vi "Activate License throuch Network.vi"() -> ()   [LabVIEW 2018]
doc: "Demonstrates how to activate a license through network api."
panel:
  out "is permanent":bool
  out "is runtime":bool
  out "days":i32
  out "result":i8
  in  "License Key":string
  in  "License ID":string="300031"
  in  "product":string="openvino"
  # "Overview: Demonstrates how to activate a license through network api.\nRequirements: Windows.\nInstructions: \n1. Fill in the product name (opencv_dnn, openvino, onnx_gpu, tensorRT and etc), License ID and License Key in the controls.\n2. Run the VI.\n3. This VI returns four information: activation success or failure, usage days(network temporary version) , whether it is a permanent version, and whether it is a runtime deployment version."
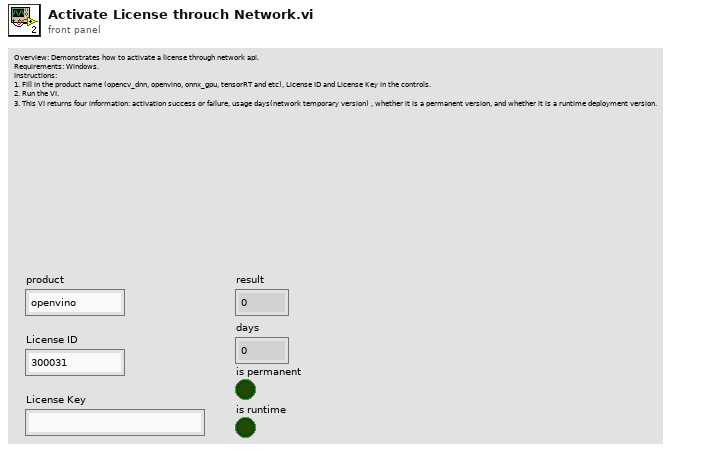
[diagram p1: front panel]
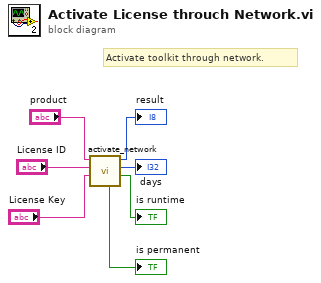
[diagram p0: block diagram]
diagram:
  # "Activate toolkit through network."
  n1 = call "activate_network.vi"("licensekey"="License Key", "licenseid"="License ID", "product"="product") -> ("is runtime"=→"is runtime":bool, "days"=→"days":i32, "result"=→"result":i8, "is permanent"=→"is permanent":bool)  [unwired: 4 in, 1 out]
